vi "build_array_activity_20.vi"() -> ()   [LabVIEW 2025]
panel:
  out "1D array":i32[](array[numeric])
  in  "Array 2":i32[](array[numeric])
  in  "scalar 3":i32
  in  "scalar 2":i32
  in  "scalar 1":i32
  in  "Array 1":i32[](array[numeric])
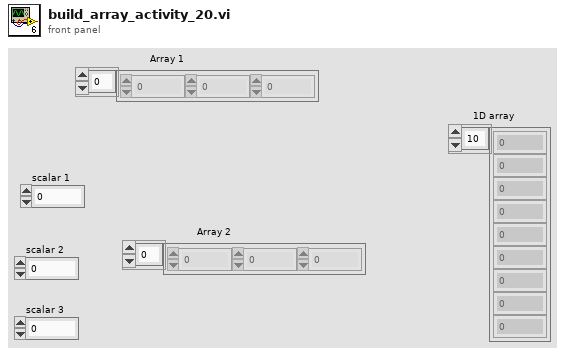
[diagram p1: front panel]
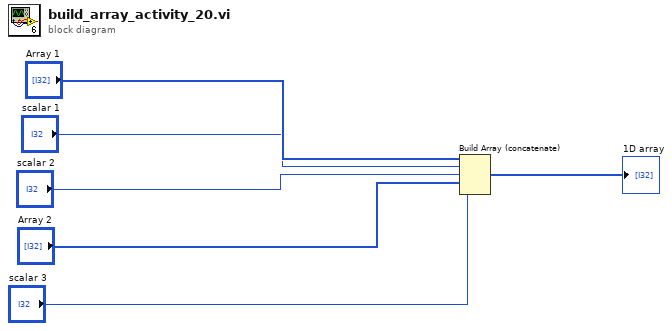
[diagram p0: block diagram]
diagram:
  n1 = Build Array (concatenate)("Array 1", "scalar 1", "scalar 2", "Array 2", "scalar 3") -> (→"1D array":i32[])
